vi "Globle.vi"() -> ()   [LabVIEW 2015]
panel:
  out "进度条":bool
  out "行号":u32
  in  "保存路径":path
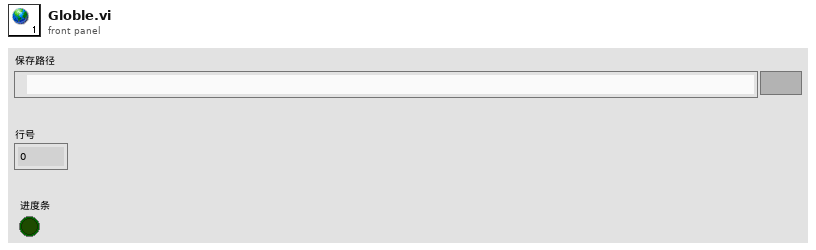
[diagram p1: front panel]
diagram:
